vi "Evaluate Jacobian.vi"(1 "m":i32, 2 "Point (x_1, ..., x_n)":dbl[](array[numeric]), 4 "Function Reference":refnum<vi>) -> (0 "Df(x)":dbl[][](array[numeric]))   [LabVIEW 2020, in "Automatic Differentiation.lvlib"]
uses:
  Automatic Differentiation.lvlib
  classes/Dual/Dual.lvclass
  classes/Dual/Dual.lvclass/Dual.ctl
  d3fc5611-aad1-4343-aaaf-f0a6943ff05c.vi
  d3fc5611-aad1-4343-aaaf-f0a6943ff05c.vi/5957e011-cf56-4527-b6ed-13c3a4ca997b.vi
  classes/Dual/Write a.vi
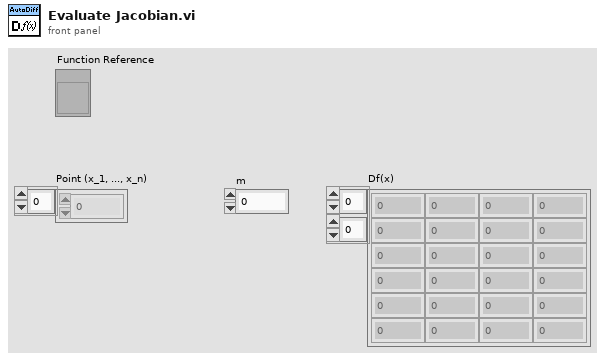
[diagram p1: front panel]
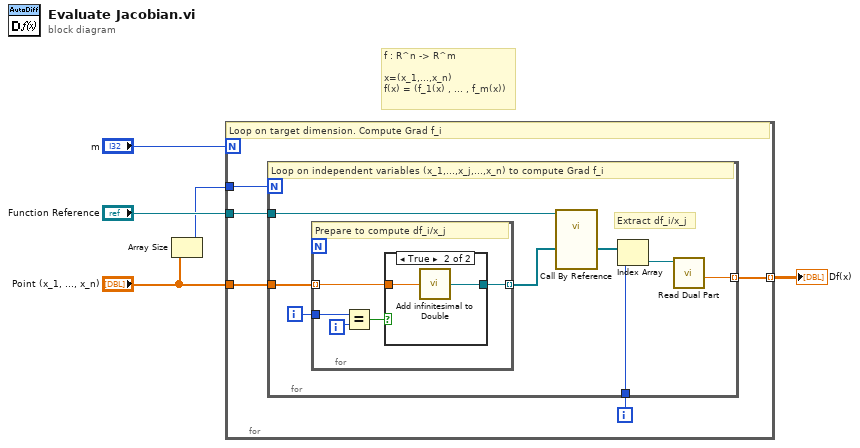
[diagram p0: block diagram]
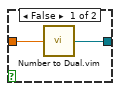
[diagram p2: hidden frame]
diagram:
  # "f : R^n -> R^m\n\nx=(x_1,...,x_n)\nf(x) = (f_1(x) , ... , f_m(x))"
  n1 = Array Size(array="Point (x_1, ..., x_n)") -> (size(s)=w3:i32)
  n2 = for {
    N: "m" -> [_]
    tunnel: "Function Reference" -> [w10]
    tunnel: "Point (x_1, ..., x_n)" -> [w9]
    tunnel: w3 -> [w8]
    tunnel: [w6] -> w1 mode=indexing
    i -> [w7]
    # "Loop on target dimension. Compute Grad f_i"
    n3 = for {
      N: w8 -> [_]
      tunnel: w10 -> [w18]
      tunnel: w9 -> [w15]
      tunnel: [w11] -> w6 mode=indexing
      tunnel: w7 -> [w13]
      i -> [w14]
      # "Extract df_i/x_j"
      # "Loop on independent variables (x_1,...,x_j,...,x_n) to compute Grad f_i"
      n4 = for {
        tunnel: w14 -> [w23]
        tunnel: w15 -> [w21] mode=indexing
        tunnel: [w19] -> w16 mode=indexing
        i -> [w22]
        # "Prepare to compute df_i/x_j"
        n5 = Equal?(x=w23, y=w22) -> (x = y?=w20:bool)
        n6 = case shown="True" w20 {
          tunnel: w21 -> [w25 w27]
          tunnel: [w24 w26] -> w19
          frame False {
            n7 = call "Number to Dual.vim"("Number"=w25) -> ("Dual"=w24:refnum<class "Dual.lvclass">)
          }
          frame True {
            n8 = call "Add infinitesimal to Double.vi"("DBL (x)"=w27) -> ("Dual (x+e)"=w26:refnum<class "Dual.lvclass">)
          }
        }
      }
      n9 = call-by-ref "?"(reference=w18, "(x_1,...,x_n)"=w16) -> ("(f_1,...,f_n)"=w17:refnum<class "Dual.lvclass">[])  [unwired: 1 in, 2 out]
      n10 = Index Array(array=w17, index=w13) -> (element=w12:refnum<class "Dual.lvclass">)
      n11 = call "Read Dual Part.vi"("Dual in"=w12) -> ("Dual Part"=w11:dbl)  [unwired: 9 in, 1 out]
    }
  }
  "Df(x)" <- w1
